vi "Teleop.vi"(10 "Match Info":T1={"Autonomous Elapsed Seconds"=0.0, "TeleOp Elapsed Seconds"=0.0, "Disabled Elapsed Seconds"=0.0, "Visited Autonomous"=FALSE, "Visited TeleOp"=FALSE, "Visited Disabled"=FALSE, "Autonomous Settings"={"Autonomous Style"=enum."Independent", "VI Refnum"=refnum}}, 11 "Call Context":T2) -> ()   [LabVIEW 2015]
doc: "This VI is called for each TeleOp packet received from the DS where the robot is not disabled. It is often used to read from the joysticks and update I/O or to update setpoints for timed control loops. It should complete and return within 20 milliseconds or it may miss DS packets."
uses:
  <vilib>/Rock Robotics/WPI/DriverStation/WPI_DriverStationDerivedRobotMode.ctl
  <vilib>/Rock Robotics/WPI/DriverStation/WPI_DriverStationMatch Info.ctl
  <vilib>/Rock Robotics/Network Tables/NT Read Boolean.vi
  <vilib>/Rock Robotics/Network Tables/NT Read Number.vi
  <vilib>/Rock Robotics/WPI/Utilities/WPI_GetSetVariantRefNum.vi
  <vilib>/Rock Robotics/Network Tables/SD Write Number.vi
  <vilib>/Rock Robotics/Network Tables/SD Write Boolean.vi
  navX Library v2/navX Library v2.lvlib
panel:
  out "Displacement X":dbl
  out "Velocity X":dbl
  out "Sample Slider 0":dbl(slide) scale=0.0..5.0
  out "Sample Boolean 1":bool
  out "Sample Boolean 0":bool
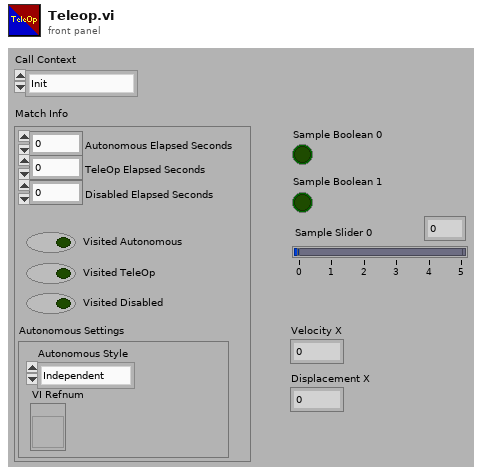
[diagram p1: front panel]
types:
  T1 = typedef "WPI_DriverStationMatch Info.ctl" = cluster{"Autonomous Elapsed Seconds":dbl, "TeleOp Elapsed Seconds":dbl, "Disabled Elapsed Seconds":dbl, "Visited Autonomous":bool, "Visited TeleOp":bool, "Visited Disabled":bool, "Autonomous Settings":cluster{"Autonomous Style":enum16{"Iterative", "Independent"}, "VI Refnum":refnum<vi>}}
  T2 = typedef "WPI_DriverStationDerivedRobotMode.ctl" = enum16{"Init", "Execute", "Stop"}
  T3 = typedef "navX Library v2.lvlib/Z900_navX_DeviceTypeDef.ctl" = cluster{"Interface":cluster{"Protocol":T4, "Update Rate (4Hz-60Hz)":u8, "navX Open TypeDef":variant}, "Notify Packet":refnum<notifier>, "Loop VI Refnum":refnum<vi>, "Ready to Close Occurrence Refnum":refnum<k4>}
  T4 = typedef "navX Library v2.lvlib/Z900_navX_ProtocolTypeDef.ctl" = enum16{"SERIAL", "I2C", "SPI"}
  T5 = typedef "WPI_JoystickDevRef.ctl" = cluster{"Device":T6}
  T6 = typedef "WPI_JoystickDeviceEnum.ctl" = enum16{"USB 0", "USB 1", "USB 2", "USB 3", "USB 4", "USB 5"}
  T7 = cluster{"Velocity X":dbl, "Velocity Y":dbl, "Velocity Z":dbl, "Displacement X":dbl, "Displacement Y":dbl, "Displacement Z":dbl}
  T8 = cluster{"Axes[0]":dbl, "Axes[1]":dbl, "Axes[2]":dbl, "Axes[3]":dbl, "Axes[4]":dbl, "Axes[5]":dbl, "Axes[6]":dbl, "Axes[7]":dbl, "Axes[8]":dbl}
  T9 = cluster{"Buttons[0]":bool, "Buttons[1]":bool, "Buttons[2]":bool, "Buttons[3]":bool, "Buttons[4]":bool, "Buttons[5]":bool, "Buttons[6]":bool, "Buttons[7]":bool, "Buttons[8]":bool}
  T10 = typedef "WPI_EncoderDevRef.ctl" = cluster{"DevStatus":errorcluster, "EncoderIndex":T11, "CounterIndex":T12, "DistancePerCount":dbl, "Decoding Type":T13}
  T11 = typedef "FPGA_EncoderIdx.ctl" = enum8{"Enc 0", "Enc 1", "Enc 2", "Enc 3", "Enc 4", "Enc 5", "Enc 6", "Enc 7", "Invalid"}
  T12 = typedef "FPGA_CounterCtrSystemIndex.ctl" = enum8{"Ctr 0", "Ctr 1", "Ctr 2", "Ctr 3", "Ctr 4", "Ctr 5", "Ctr 6", "Ctr 7", "Invalid"}
  T13 = typedef "WPI_EncoderType.ctl" = enum16{"1x", "2x", "4x"}
  T14 = typedef "WPI_RobotDriveDevRef.ctl" = cluster{"DevStatus":errorcluster, "Motors[]":T15[], "Square Inputs":bool, "Max Output":dbl}
  T15 = typedef "WPI_MotorControlDeviceRef.ctl" = cluster{"DeviceStatus":errorcluster, "Type":T16, "PWM":cluster{"PWM Channel":T17, "DeadBand":T18}, "CAN":cluster{"Device Number":u8, "Control Mode":T19, "Semaphore":T20, "Max Vout":dbl, "TalonSRX Control Mode":T21}, "Invert":bool}
  T16 = typedef "WPI_MotorControlType.ctl" = enum16{"PWM", "CAN", "CANTalonSRX"}
  T17 = typedef "FPGA_DIOPWMChannel.ctl" = enum8{"PWM 0", "PWM 1", "PWM 2", "PWM 3", "PWM 4", "PWM 5", "PWM 6", "PWM 7", "PWM 8", "PWM 9", "PWM MXP 0", "PWM MXP 1", "PWM MXP 2", "PWM MXP 3", "PWM MXP 4", "PWM MXP 5", "PWM MXP 6", "PWM MXP 7", "PWM MXP 8", "PWM MXP 9", "Invalid"}
  T18 = typedef "WPI_PWMDeadband.ctl" = cluster{"Name":string, "maxPositivePwm":i32, "minPositivePwm":i32, "centerPwm":i32, "maxNegativePwm":i32, "minNegativePwm":i32, "angularRange":u16}
  T19 = typedef "WPI_CANJaguar_ControlMode.ctl" = enum8{"Percent VBus", "Current", "Speed", "Position", "Voltage"}
  T20 = typedef "Semaphore RefNum" = refnum<k1>
  T21 = typedef "WPI_CANTalonSRX_APIControlMode.ctl" = enum8{"Percent VBus", "Speed", "Position", "Slave", "Unchanged / Invalid", "Voltage Compensation", "Current", "Motion Profile"}
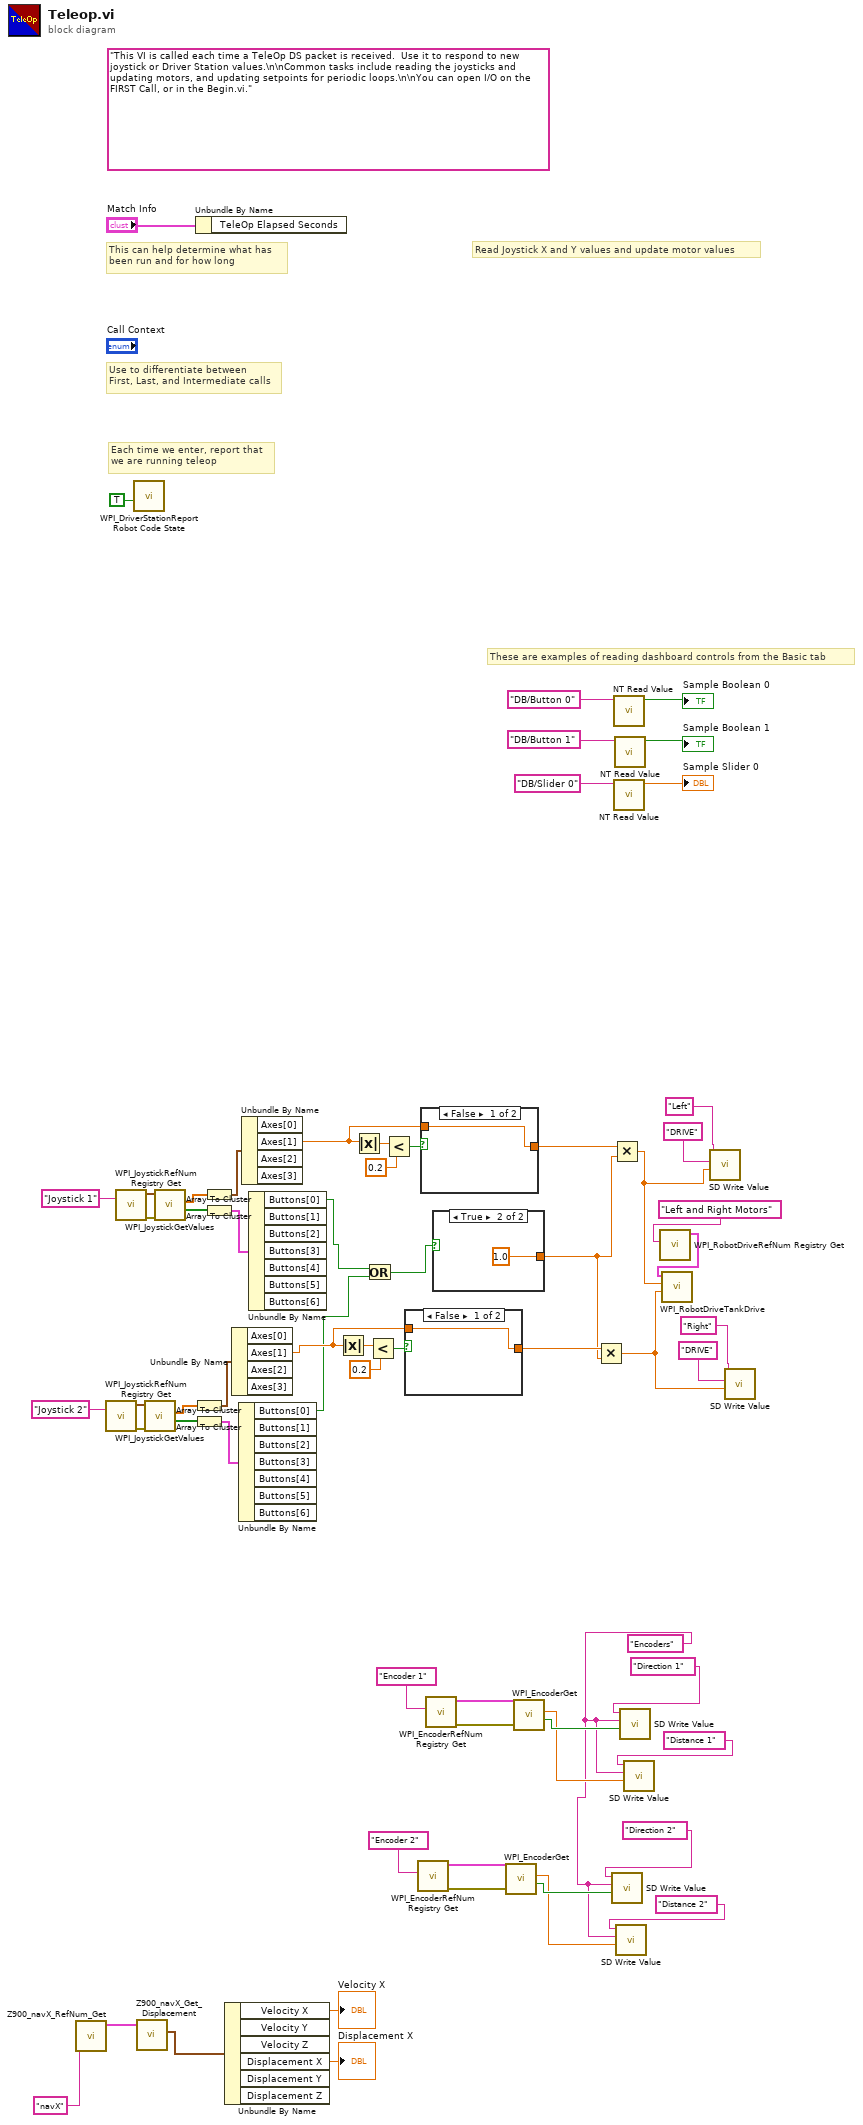
[diagram p0: block diagram]
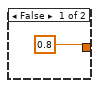
[diagram p2: hidden frame]
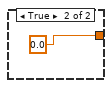
[diagram p3: hidden frame]
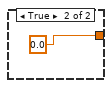
[diagram p4: hidden frame]
diagram:
  w6 = "Encoders"
  (unwired) "This VI is called each time a TeleOp DS packet is received.  Use it to respond to new joystick or Driver Station values.\n\nCommon tasks include reading the joysticks and updating motors, and updating setpoints for periodic loops.\n\nYou can open I/O on the FIRST Call, or in the Begin.vi."
  # "These are examples of reading dashboard controls from the Basic tab"
  # "Each time we enter, report that\nwe are running teleop"
  # "Use to differentiate between\nFirst, Last, and Intermediate calls"
  # "This can help determine what has\nbeen run and for how long"
  # "Read Joystick X and Y values and update motor values"
  n1 = call "Z900_navX_RefNum_Get.vi"("refnum name"="navX") -> ("navX Device"=w5:T3)  [unwired: 9 in, 1 out]
  n2 = call <vilib>:"WPI_JoystickRefNum Registry Get.vi"("refnum name"="Joystick 2") -> ("error out"=w48:errorcluster, "JoystickDevRef"=w47:T5)  [unwired: 9 in]
  n3 = call <vilib>:"WPI_JoystickRefNum Registry Get.vi"("refnum name"="Joystick 1") -> ("error out"=w55:errorcluster, "JoystickDevRef"=w54:T5)  [unwired: 9 in]
  n4 = call <vilib>:"WPI_DriverStationReport Robot Code State.vi"("TeleOp"=TRUE ("Autonomous")) -> ()  [unwired: 10 in, 1 out]
  n5 = call "Z900_navX_Get_Displacement.vi"("navX Device"=w5) -> ("Displacement"=w3:T7)  [unwired: 7 in, 3 out]
  n6 = call <vilib>:"WPI_JoystickGetValues.vi"("error in (no error)"=w48, "JoystickDevRef"=w47) -> ("Buttons"=w45:bool[], "Axes"=w46:dbl[])  [unwired: 5 in, 3 out]
  n7 = call <vilib>:"WPI_JoystickGetValues.vi"("error in (no error)"=w55, "JoystickDevRef"=w54) -> ("Buttons"=w52:bool[], "Axes"=w53:dbl[])  [unwired: 5 in, 3 out]
  n8 = Array To Cluster(array=w46) -> (cluster=w44:T8)
  n9 = Array To Cluster(array=w45) -> (cluster=w43:T9)
  n10 = Unbundle By Name("Match Info") -> ()  [unwired: 1 out]
  n11 = Array To Cluster(array=w53) -> (cluster=w51:T8)
  n12 = Array To Cluster(array=w52) -> (cluster=w50:T9)
  n13 = Unbundle By Name(w3) -> ("Velocity X"=→"Velocity X":dbl, "Displacement X"=→"Displacement X":dbl)  [unwired: 4 out]
  n14 = Unbundle By Name(w44) -> ("Axes[1]"=w33:dbl)  [unwired: 3 out]
  n15 = Unbundle By Name(w43) -> ("Buttons[0]"=w22:bool)  [unwired: 6 out]
  n16 = Unbundle By Name(w51) -> ("Axes[1]"=w38:dbl)  [unwired: 3 out]
  n17 = Unbundle By Name(w50) -> ("Buttons[0]"=w23:bool)  [unwired: 6 out]
  n18 = Absolute Value(x=w33) -> (abs(x)=w37:dbl)
  n19 = Absolute Value(x=w38) -> (abs(x)=w42:dbl)
  n20 = Or(x=w23, y=w22) -> (x .or. y?=w21:bool)
  n21 = Less?(x=w37, y=0.2) -> (x < y?=w35:bool)
  n22 = Less?(x=w42, y=0.2) -> (x < y?=w40:bool)
  n23 = case shown="False" w35 {
    tunnel: [w65 0.0] -> w34
    tunnel: w33 -> [w65 _]
    frame False {
    }
    frame True {
    }
  }
  n24 = call <vilib>:"WPI_EncoderRefNum Registry Get.vi"("refnum name"="Encoder 2") -> ("error out"=w12:errorcluster, "EncoderDevRef"=w11:T10)  [unwired: 9 in]
  n25 = case shown="False" w40 {
    tunnel: [w67 0.0] -> w39
    tunnel: w38 -> [w67 _]
    frame False {
    }
    frame True {
    }
  }
  n26 = call <vilib>:"WPI_EncoderRefNum Registry Get.vi"("refnum name"="Encoder 1") -> ("error out"=w19:errorcluster, "EncoderDevRef"=w18:T10)  [unwired: 9 in]
  n27 = case shown="True" w21 {
    tunnel: [0.8 1.0] -> w32
    frame False {
    }
    frame True {
    }
  }
  n28 = call <vilib>:"WPI_EncoderGet.vi"("error in (no error)"=w12, "EncoderDevRef"=w11) -> ("Direction"=w10:bool, "Distance"=w8:dbl)  [unwired: 4 in, 4 out]
  n29 = call <vilib>:"WPI_EncoderGet.vi"("error in (no error)"=w19, "EncoderDevRef"=w18) -> ("Direction"=w17:bool, "Distance"=w15:dbl)  [unwired: 4 in, 4 out]
  n30 = Multiply(x=w34, y=w32) -> (x*y=w27:dbl)
  n31 = Multiply(x=w39, y=w32) -> (x*y=w24:dbl)
  n32 = call-poly <vilib>:"SD Write Value.vi"("Boolean"=w10, "Table Prefix"=w6, "Name"="Direction 2") -> ()  [unwired: 7 in, 2 out]
  n33 = call-poly <vilib>:"NT Read Value.vi"("Name"="DB/Button 0" ("refnum name")) -> ("Boolean"=→"Sample Boolean 0":bool)  [unwired: 9 in, 1 out]
  n34 = call-poly <vilib>:"NT Read Value.vi"("Name"="DB/Slider 0" ("refnum name")) -> ("Numeric"=→"Sample Slider 0":dbl)  [unwired: 9 in, 1 out]
  n35 = call-poly <vilib>:"NT Read Value.vi"("Name"="DB/Button 1" ("refnum name")) -> ("Boolean"=→"Sample Boolean 1":bool)  [unwired: 9 in, 1 out]
  n36 = call-poly <vilib>:"SD Write Value.vi"("Numeric"=w8, "Table Prefix"=w6, "Name"="Distance 2") -> ()  [unwired: 7 in, 2 out]
  n37 = call-poly <vilib>:"SD Write Value.vi"("Boolean"=w17, "Table Prefix"=w6, "Name"="Direction 1") -> ()  [unwired: 7 in, 2 out]
  n38 = call-poly <vilib>:"SD Write Value.vi"("Numeric"=w15, "Table Prefix"=w6, "Name"="Distance 1") -> ()  [unwired: 7 in, 2 out]
  n39 = call <vilib>:"WPI_RobotDriveRefNum Registry Get.vi"("refnum name"="Left and Right Motors") -> ("RobotDriveDevRef"=w31:T14)  [unwired: 9 in, 1 out]
  n40 = call <vilib>:"WPI_RobotDriveTankDrive.vi"("Right axis value"=w27, "Left axis value"=w24, "RobotDriveDevRef"=w31) -> ()  [unwired: 6 in, 3 out]
  n41 = call-poly <vilib>:"SD Write Value.vi"("Numeric"=w24, "Table Prefix"="DRIVE", "Name"="Left") -> ()  [unwired: 7 in, 2 out]
  n42 = call-poly <vilib>:"SD Write Value.vi"("Numeric"=w27, "Table Prefix"="DRIVE", "Name"="Right") -> ()  [unwired: 7 in, 2 out]
